vi "Write was run.vi"(8 "error in (no error)":errorcluster, 10 "was run":bool, 11 "WasRun in":refnum<class "WasRun.lvclass">) -> (0 "error out":errorcluster, 3 "WasRun out":refnum<class "WasRun.lvclass">)   [LabVIEW 2013, in "WasRun.lvclass"]
uses:
  WasRun.lvclass
  WasRun.lvclass/WasRun.ctl
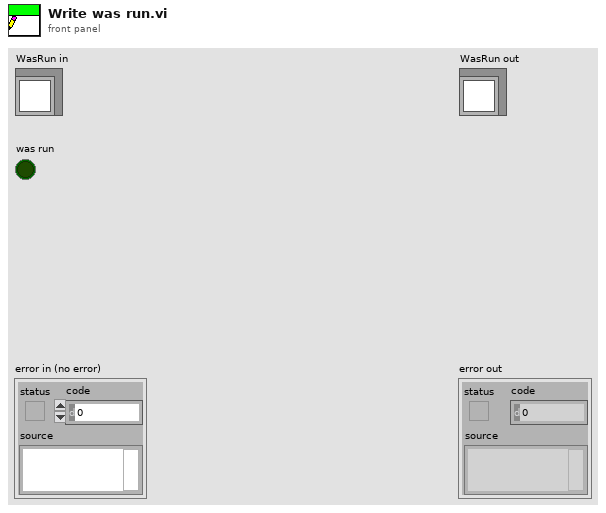
[diagram p1: front panel]
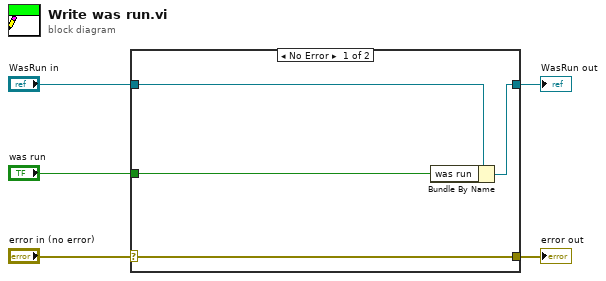
[diagram p0: block diagram]
diagram:
  n1 = case shown="No Error" "error in (no error)" {
    selector: "error in (no error)" -> [w9 w10]
    tunnel: [w9 w10] -> w4
    tunnel: [w7 w11] -> w2
    tunnel: "WasRun in" -> [w8 w11]
    tunnel: "was run" -> [w6 _]
    frame No Error {
      n2 = Bundle By Name(cluster=w8, "was run"=w6) -> (w7:refnum<class "WasRun.lvclass">)
    }
    frame Error {
    }
  }
  "error out" <- w4
  "WasRun out" <- w2
